vi "trans_time.vi"(10 "Numeric":i32) -> (2 "time":string)   [LabVIEW 2012]
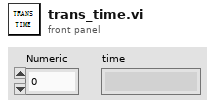
[diagram p1: front panel]
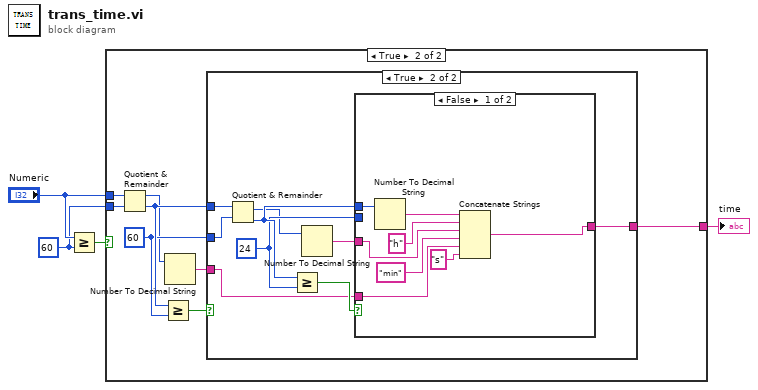
[diagram p0: block diagram]
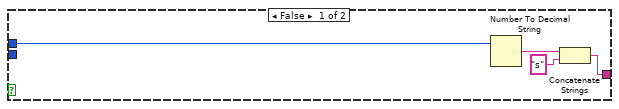
[diagram p2: hidden frame]
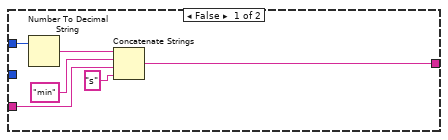
[diagram p3: hidden frame]
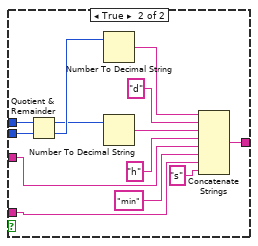
[diagram p4: hidden frame]
diagram:
  w2 = 60 ("y")
  n1 = Greater Or Equal?(x="Numeric", y=w2) -> (x >= y?=w4:bool)
  n2 = case shown="True" w4 {
    tunnel: "Numeric" -> [w8 w14]
    tunnel: [w5 w9] -> w1
    tunnel: w2 -> [_ w15]
    frame False {
      n3 = Number To Decimal String(number=w8) -> (decimal integer string=w7:string)  [unwired: 1 in]
      n4 = Concatenate Strings(w7, "s" ("string")) -> (w5:string)
    }
    frame True {
      w12 = 60 ("y")
      n5 = Quotient & Remainder(x=w14, y=w15) -> (x-y*floor(x/y)=w11:i32, floor(x/y)=w13:i32)
      n6 = Greater Or Equal?(x=w13, y=w12) -> (x >= y?=w16:bool)
      n7 = Number To Decimal String(number=w11) -> (decimal integer string=w10:string)  [unwired: 1 in]
      n8 = case shown="True" w16 {
        tunnel: w13 -> [w22 w31]
        tunnel: w12 -> [_ w27]
        tunnel: w10 -> [w19 w24]
        tunnel: [w17 w23] -> w9
        frame False {
          n9 = Number To Decimal String(number=w22) -> (decimal integer string=w21:string)  [unwired: 1 in]
          n10 = Concatenate Strings(w21, "min" ("string"), w19, "s" ("string")) -> (w17:string)
        }
        frame True {
          w28 = 24 ("y")
          n11 = Quotient & Remainder(x=w31, y=w27) -> (x-y*floor(x/y)=w26:i32, floor(x/y)=w29:i32)
          n12 = Greater Or Equal?(x=w29, y=w28) -> (x >= y?=w30:bool)
          n13 = Number To Decimal String(number=w26) -> (decimal integer string=w25:string)  [unwired: 1 in]
          n14 = case shown="False" w30 {
            tunnel: w29 -> [w39 w52]
            tunnel: w28 -> [_ w51]
            tunnel: w25 -> [w36 w44]
            tunnel: w24 -> [w34 w42]
            tunnel: [w32 w40] -> w23
            frame False {
              n15 = Number To Decimal String(number=w39) -> (decimal integer string=w38:string)  [unwired: 1 in]
              n16 = Concatenate Strings(w38, "h" ("string"), w36, "min" ("string"), w34, "s" ("string")) -> (w32:string)
            }
            frame True {
              n17 = Quotient & Remainder(x=w52, y=w51) -> (x-y*floor(x/y)=w47:i32, floor(x/y)=w50:i32)
              n18 = Number To Decimal String(number=w50) -> (decimal integer string=w49:string)  [unwired: 1 in]
              n19 = Number To Decimal String(number=w47) -> (decimal integer string=w46:string)  [unwired: 1 in]
              n20 = Concatenate Strings(w49, "d" ("string"), w46, "h" ("string"), w44, "min" ("string"), w42, "s" ("string")) -> (w40:string)
            }
          }
        }
      }
    }
  }
  "time" <- w1
